vi "emi_Defer Panel Updates ON.vi"(5 "VI Refnum(This VI)":refnum<vi>, 9 "error in (no error)":errorcluster) -> (6 "VI Refnum Out":refnum<vi>, 10 "error out":errorcluster)   [LabVIEW 2011]
doc: "Gets a vi panel refrence, sets defere panel update to true, close panel refrence.\n\nIf not VI Refnum in, the refrence of the vi where this funciton is used is employed, and subsequently closed. (If refrence not explisitly vired, it does not need to be closed)\n\nIf error: No action."
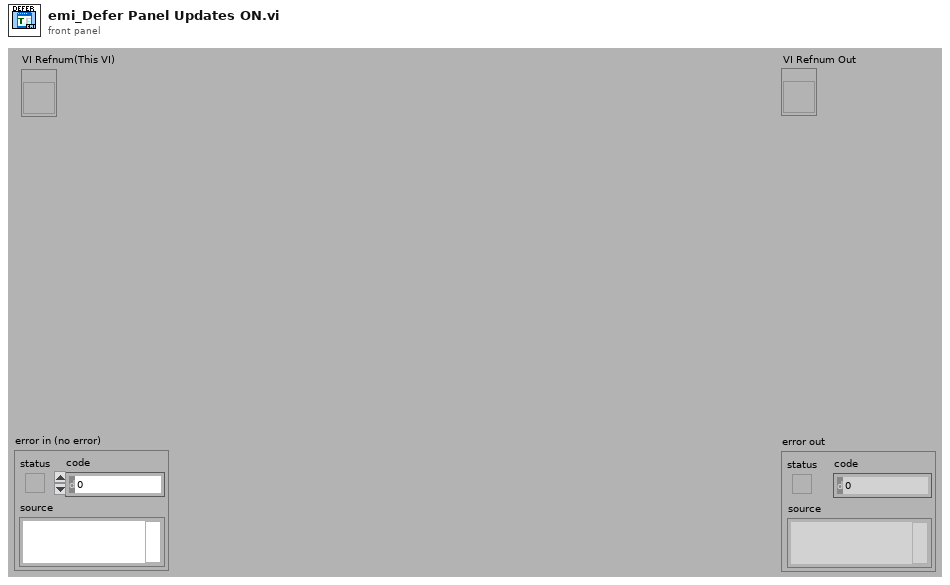
[diagram p1: front panel]
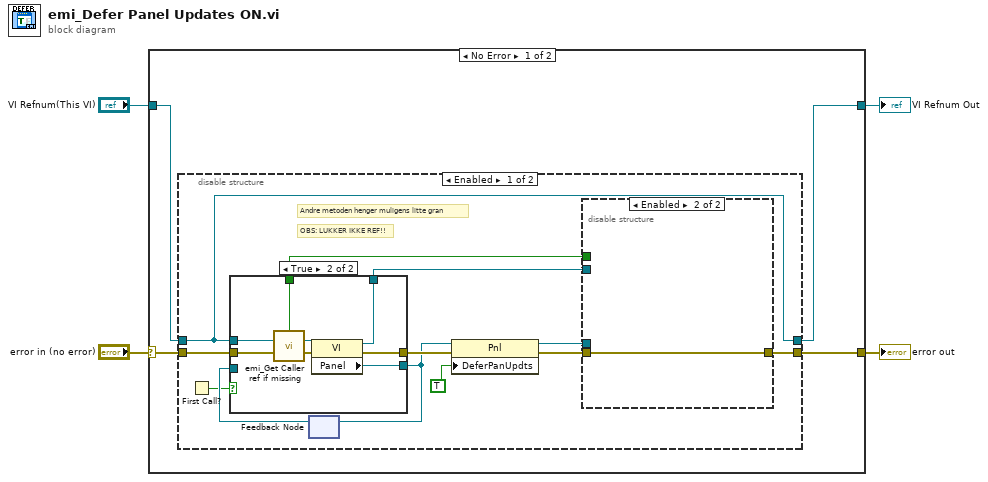
[diagram p0: block diagram]
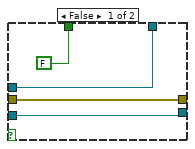
[diagram p2: hidden frame]
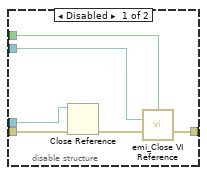
[diagram p3: hidden frame]
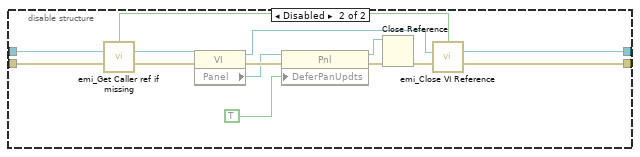
[diagram p4: hidden frame]
diagram:
  n1 = case shown="No Error" "error in (no error)" {
    selector: "error in (no error)" -> [w8 w55]
    tunnel: [w7 w55] -> w3
    tunnel: "VI Refnum(This VI)" -> [w5 w54]
    tunnel: [w6 w54] -> w1
    frame No Error {
      n2 = disable-structure shown="Enabled" {
        disable-tunnel: w8 -> [w15 w47]
        disable-tunnel: [w14 w45] -> w7
        disable-tunnel: [w12 w41] -> w6
        disable-tunnel: w5 -> [w12 w40]
        frame Enabled {
          # "OBS: LUKKER IKKE REF!!"
          # "Andre metoden henger muligens litte gran"
          n3 = First Call?() -> (First Call?: T/F=w9:bool)
          n4 = feedback #1() -> (w10:refnum<vi>)  [unwired: 1 in]
          n5 = case shown="True" w9 {
            tunnel: [w24 w32] -> w19
            tunnel: [w23 w31] -> w11
            tunnel: [FALSE ("Ref Generated") w30] -> w16
            tunnel: w15 -> [w24 w29]
            tunnel: [w22 w26] -> w13
            tunnel: w12 -> [w22 w25]
            tunnel: w10 -> [w23 _]
            frame False {
            }
            frame True {
              n6 = call "emi_Get Caller ref if missing.vi"("VI Refnum(Calling VI)"=w25, "error in (no error)"=w29) -> ("Ref Generated"=w30:bool, "VI Refnum Out"=w27:refnum<vi>, "error out"=w28:errorcluster)  [unwired: 11 in]
              n7 = property class="VI"(reference=w27, error in=w28) -> (reference out=w26:refnum<vi>, error out=w32:errorcluster, "Panel"=w31:refnum<vi>)
            }
          }
          n8 = feedback-in #1(w11) -> ()
          n9 = property class="Pnl"(reference=w11, error in=w19, "DeferPanUpdts"=TRUE ("Defer Panel Updates")) -> (reference out=w18:refnum<vi>, error out=w17:errorcluster)
          n10 = disable-structure shown="Enabled" {
            disable-tunnel: w18 -> [w38 _]
            disable-tunnel: w17 -> [w37 w39]
            disable-tunnel: w16 -> [w36 _]
            disable-tunnel: [w35 w39] -> w14
            disable-tunnel: w13 -> [w33 _]
            frame Disabled {
              n11 = Close Reference(reference=w38, error in (no error)=w37) -> (error out=w34:errorcluster)
              n12 = call "emi_Close VI Reference.vi"("Close ref?(T)"=w36, "VI Refnum"=w33, "error in (no error)"=w34) -> ("error out"=w35:errorcluster)  [unwired: 11 in, 1 out]
            }
            frame Enabled {
            }
          }
        }
        frame Disabled {
          n13 = call "emi_Get Caller ref if missing.vi"("VI Refnum(Calling VI)"=w40, "error in (no error)"=w47) -> ("Ref Generated"=w48:bool, "VI Refnum Out"=w43:refnum<vi>, "error out"=w46:errorcluster)  [unwired: 11 in]
          n14 = property class="VI"(reference=w43, error in=w46) -> (reference out=w42:refnum<vi>, error out=w52:errorcluster, "Panel"=w51:refnum<vi>)
          n15 = property class="Pnl"(reference=w51, error in=w52, "DeferPanUpdts"=TRUE ("Defer Panel Updates")) -> (reference out=w50:refnum<vi>, error out=w49:errorcluster)
          n16 = Close Reference(reference=w50, error in (no error)=w49) -> (error out=w44:errorcluster)
          n17 = call "emi_Close VI Reference.vi"("Close ref?(T)"=w48, "VI Refnum"=w42, "error in (no error)"=w44) -> ("VI Refnum Out"=w41:refnum<vi>, "error out"=w45:errorcluster)  [unwired: 11 in]
        }
      }
    }
    frame Error {
    }
  }
  "error out" <- w3
  "VI Refnum Out" <- w1
